vi "test_turbo3.vi"() -> ()   [LabVIEW 2018]
uses:
  <vilib>/addons/Modulation/Digital/Support/Common/Validators/mod_AWGN Validate.vi
  <vilib>/addons/Modulation/Analog/support/mod_Set Error Source.vi
  <vilib>/addons/Modulation/Digital/Impairments/subVIs/mod_createSeeds.vi
  <vilib>/addons/Modulation/Digital/Support/Common/Validators/mod_Validate Samples Per Symbol.vi
  <vilib>/addons/Modulation/Analog/support/Validators/mod_Validate Complex Waveform.vi
  <vilib>/addons/Modulation/Analog/support/Validators/mod_WFErrorHandler.vi
  <vilib>/addons/Modulation/Digital/General/subVIs/mod_Generate Bits PN Sequence.vi
  <vilib>/Analysis/1siggen.llb/Gaussian White Noise (obs 90).vi
  <vilib>/addons/Modulation/Digital/General/MT Apply Matched Filter (Generic).vi
  <vilib>/addons/Modulation/niDMT.lvlib
panel:
  out "#err":i32
  in  "#trials":i32
  out "#bits":i32
  in  "Eb/N0":dbl=10.0 format="%.2f"
  out "BER":dbl
  out "Dec":i8[](array[numeric])
  out "sigma2":string
  out "trial":i32
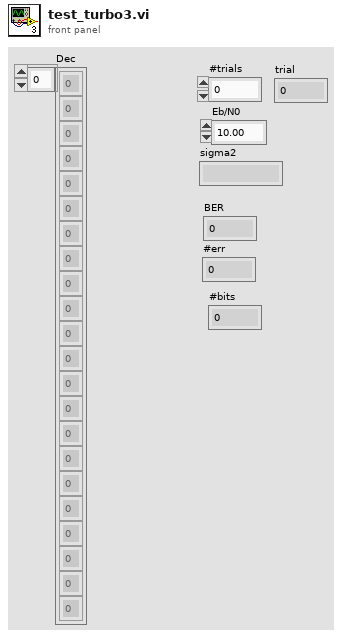
[diagram p1: front panel]
types:
  T1 = typedef "niAMT.lvlib/Complex Data Waveform.ctl" = cluster{"t0":dbl, "dt":dbl, "Y":cdb[]}
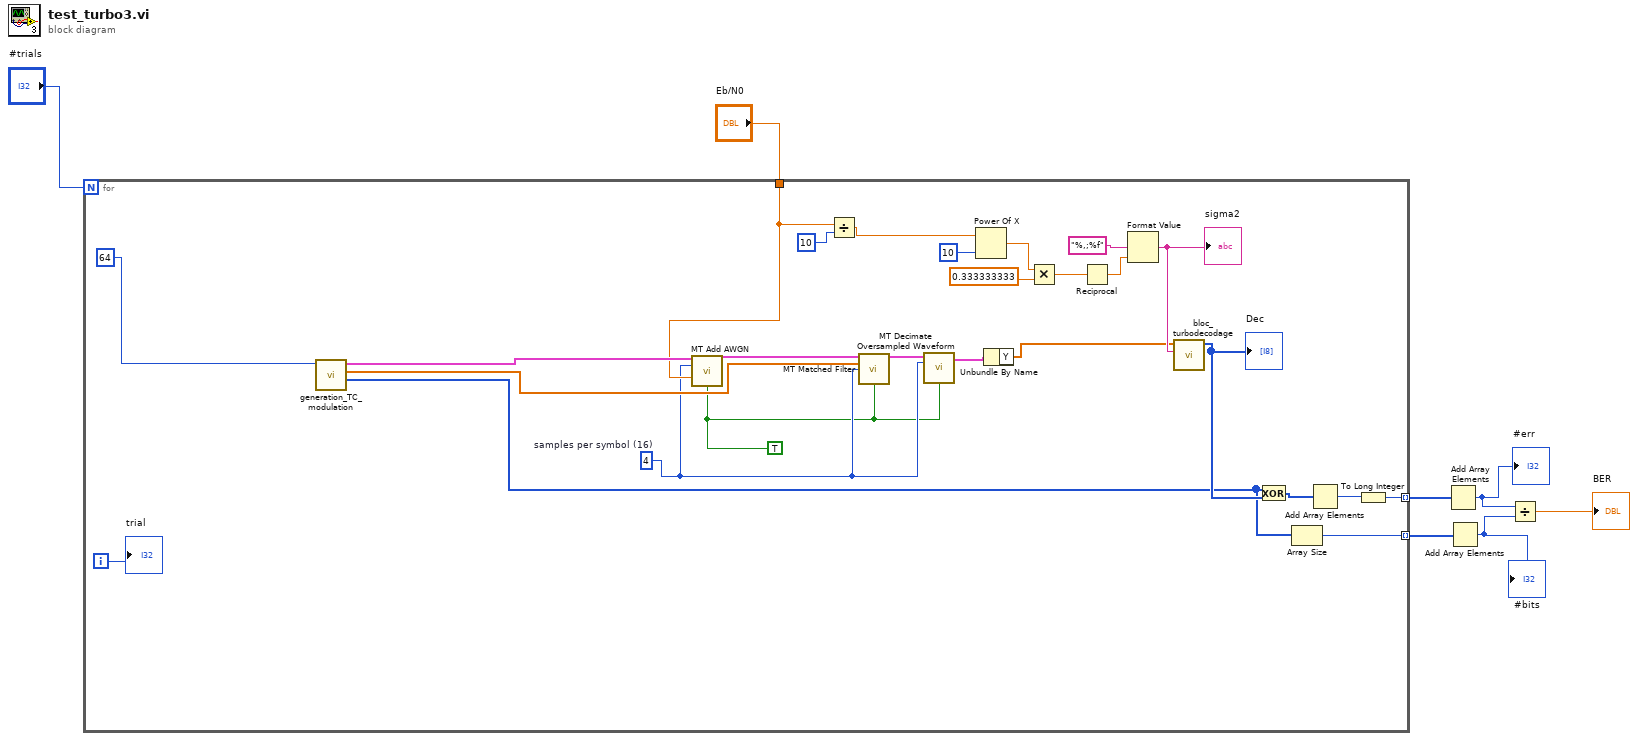
[diagram p0: block diagram]
diagram:
  n1 = for {
    N: "#trials" -> [_]
    tunnel: [w28] -> w6 mode=indexing
    tunnel: "Eb/N0" -> [w12]
    tunnel: [w19] -> w2 mode=indexing
    i -> [w21]
    w9 = 4  # samples per symbol (16)
    w8 = TRUE ("reset? (T)")
    n2 = call "generation_TC_modulation.vi"("Numeric"=64) -> ("output bit stream"=w10:i8[], "matched filter coefficients"=w18:dbl[], "output complex waveform"=w17:T1)  [unwired: 8 in]
    n3 = call <vilib>:"MT Add AWGN.vi"("input complex waveform"=w17, "samples per symbol (16)"=w9, "Eb/N0 (10 dB)"=w12, "reset? (T)"=w8) -> ("output complex waveform"=w13:T1)  [unwired: 9 in, 2 out]
    n4 = Divide(x=w12, y=10) -> (x/y=w23:dbl)
    n5 = call-poly <vilib>:"MT Matched Filter.vi"("input complex waveform"=w13, "matched filter coefficients"=w18, "samples per symbol (16)"=w9, "reset? (T)"=w8) -> ("output complex waveform"=w16:T1)  [unwired: 10 in, 1 out]
    n6 = call <vilib>:"MT Decimate Oversampled Waveform.vi"("input complex waveform"=w16, "decimation factor"=w9, "reset? (T)"=w8) -> ("output complex waveform"=w14:T1)  [unwired: 11 in, 1 out]
    n7 = Power Of X(1:10, 2:w23) -> (0:w24:dbl)
    n8 = Unbundle By Name(w14) -> ("Y"=w11:cdb[])
    n9 = Multiply(x=w24, y=0.333333333) -> (x*y=w32:dbl)
    n10 = Reciprocal(x=w32) -> (1/x=w30:dbl)
    n11 = Format Value(format string="%,;%f", value (0)=w30) -> (output string=w27:string)  [unwired: 1 in]
    "sigma2" <- w27
    n12 = call "bloc_turbodecodage.vi"("sigma2"=w27, "Array"=w11) -> ("output bit stream"=w26:i8[])  [unwired: 7 in, 2 out]
    "Dec" <- w26
    n13 = Exclusive Or(1:w26, 2:w10) -> (0:w29:i8[])
    n14 = Array Size(array=w10) -> (size(s)=w28:i32)
    n15 = Add Array Elements(numeric array=w29) -> (sum=w20:i8)
    n16 = To Long Integer(number=w20) -> (32bit integer=w19:i32)
    "trial" <- w21
  }
  n17 = Add Array Elements(numeric array=w2) -> (sum=w1:i32)
  "#err" <- w1
  n18 = Add Array Elements(numeric array=w6) -> (sum=w5:i32)
  "#bits" <- w5
  n19 = Divide(x=w1, y=w5) -> (x/y=→"BER":dbl)
